vi "JSON-DBUpdate.vi"(0 "Table":string="Inventory", 2 "Column Number":string="Inventory", 5 "SQL Statement":string, 11 "error in":errorcluster, 12 "Data":string="ReplyWithAddQuery") -> (4 "Output JSON Object":string, 15 "error out":errorcluster)   [LabVIEW 2014]
panel:
  in  "Update All":bool
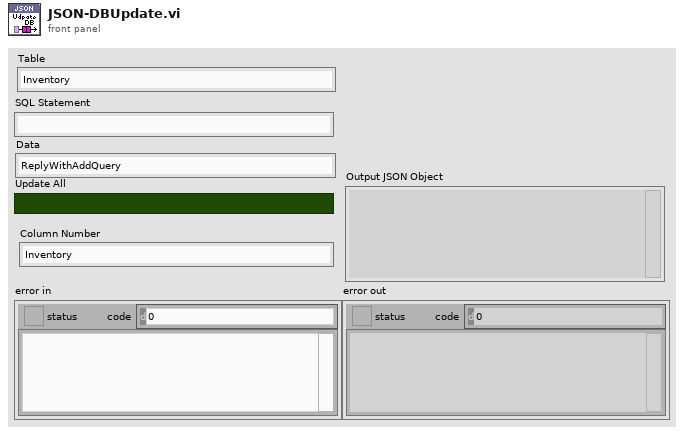
[diagram p1: front panel]
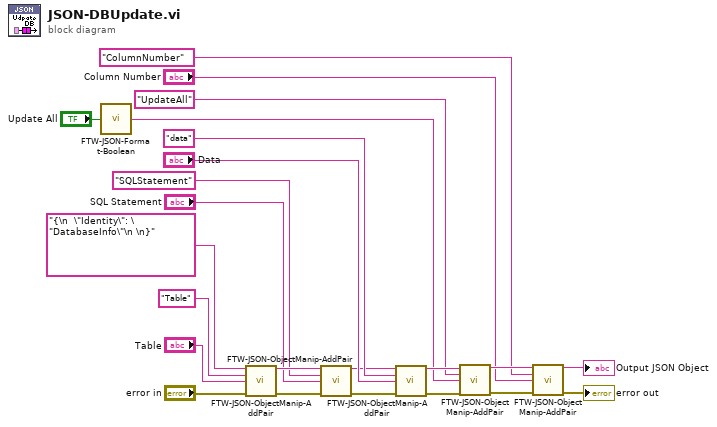
[diagram p0: block diagram]
diagram:
  n1 = call "FTW-JSON-Format-Boolean.vi"("LabVIEW Boolean"="Update All") -> ("JSON Boolean"=w2:string)
  n2 = call "FTW-JSON-ObjectManip-AddPair.vi"("Input JSON Object"="{\n  \"Identity\": \"DatabaseInfo\"\n \n}" ("FTW Actor Instance Configuration 2"), "Key"="Table", "Value"="Table", "error in"="error in") -> ("Output JSON Object"=w20:string, "error out"=w13:errorcluster)  [unwired: 10 in]
  n3 = call "FTW-JSON-ObjectManip-AddPair.vi"("Input JSON Object"=w20, "Key"="SQLStatement", "Value"="SQL Statement", "error in"=w13) -> ("Output JSON Object"=w21:string, "error out"=w12:errorcluster)  [unwired: 10 in]
  n4 = call "FTW-JSON-ObjectManip-AddPair.vi"("Input JSON Object"=w21, "Key"="data", "Value"="Data", "error in"=w12) -> ("Output JSON Object"=w11:string, "error out"=w10:errorcluster)  [unwired: 10 in]
  n5 = call "FTW-JSON-ObjectManip-AddPair.vi"("Input JSON Object"=w11, "Key"="UpdateAll", "Value"=w2, "error in"=w10) -> ("Output JSON Object"=w8:string, "error out"=w7:errorcluster)  [unwired: 10 in]
  n6 = call "FTW-JSON-ObjectManip-AddPair.vi"("Input JSON Object"=w8, "Key"="ColumnNumber", "Value"="Column Number", "error in"=w7) -> ("Output JSON Object"=→"Output JSON Object":string, "error out"=→"error out":errorcluster)  [unwired: 10 in]
